vi "FiniteMeasurement.vi"() -> ()   [LabVIEW 2022 SP3]
uses:
  controls/UI References_self.ctl
  <vilib>/Utility/miscctls.llb/LVAnnotationListTypeDef.ctl
  <vilib>/Utility/miscctls.llb/LVCursorListTypeDef.ctl
  controls/Graph Data_self.ctl
  controls/Simulated Signal Type_self.ctl
  controls/HW Configuration_self.ctl
  controls/Analysis Configuration_self.ctl
  controls/New Data Behavior_self.ctl
  controls/User Specified Data_self.ctl
  controls/Data_self.ctl
panel:
  out "状态栏":string
  out "图形":dbl[](graph)
  in  "退出":bool
  in  "导出":bool
  in  "保存":bool
  in  "复制图形":bool
  in  "分析":bool
  in  "清空":bool
  in  "加载":bool
  in  "采集":bool
  in  "设置":bool
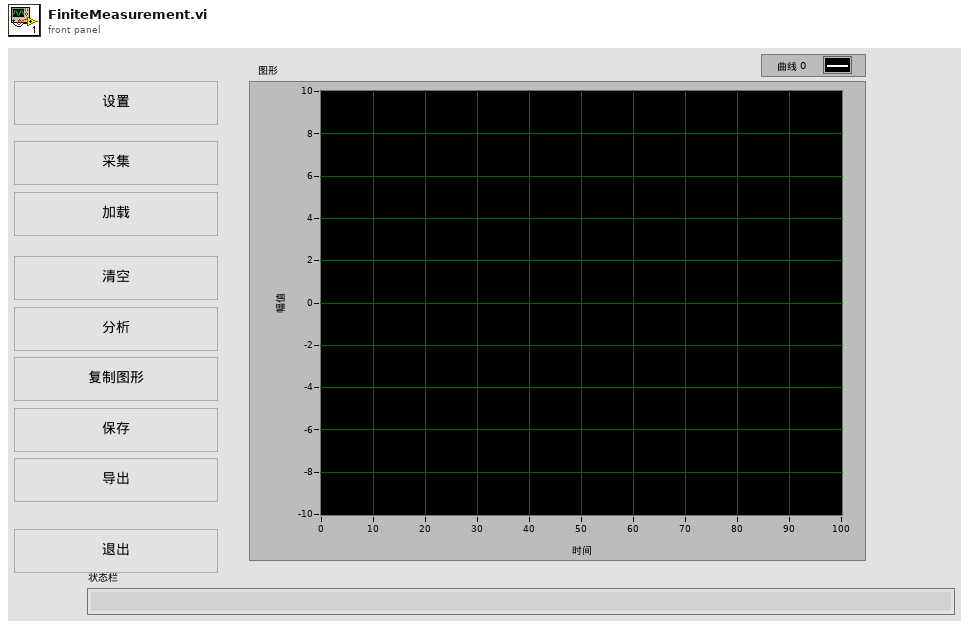
[diagram p1: front panel]
types:
  T1 = typedef "Data_self.ctl" = cluster{"UI引用":T2, "图形数据":T3, "用户定义":T6}
  T2 = typedef "UI References_self.ctl" = cluster{"退出引用":refnum<vi>, "保存引用":refnum<vi>, "打开引用":refnum<vi>, "导出引用":refnum<vi>, "采集引用":refnum<vi>, "配置引用":refnum<vi>, "图形引用":refnum<vi>, "清空引用":refnum<vi>, "分析引用":refnum<vi>, "状态引用":refnum<vi>, "快照引用":refnum<vi>}
  T3 = typedef "Graph Data_self.ctl" = cluster{"数据":waveform(dbl)[], "Annotation List":T4, "Cursor List":T5, "分析数据":waveform(dbl)[]}
  T4 = typedef "LVAnnotationListTypeDef.ctl" = cluster{"Name":string, "Color":u32, "Style":u8, "Point Style":u8, "Name Visible":bool, "Allow Drag":bool, "Annotation Mode":u32, "Plot":i32, "Index":i32, "Position":cluster{"X":dbl, "Y":dbl}, "X Scale":u32, "Y Scale":u32, "Show Arrow":bool, "Lock Name":bool, "Plot Area":i32, "Label Offset":cluster{"X":dbl, "Y":dbl}}[]
  T5 = typedef "LVCursorListTypeDef.ctl" = cluster{"Name":string, "Color":u32, "Style":u8, "Point Style":u8, "Name Visible":bool, "Allow Drag":bool, "Cursor Mode":u32, "Plot":i32, "Index":i32, "Position":cluster{"X":dbl, "Y":dbl}, "X Scale":u32, "Y Scale":u32, "Watch Plots":i32[], "Watch All Plots":bool, "Plot Area":i32, "Label Offset":cluster{"X":dbl, "Y":dbl}}[]
  T6 = typedef "User Specified Data_self.ctl" = cluster{"硬件配置":T7, "分析配置":T9, "新采集到数据时如何操作":T10}
  T7 = typedef "HW Configuration_self.ctl" = cluster{"硬件引用句柄":string, "信号类型":T8}
  T8 = typedef "Simulated Signal Type_self.ctl" = enum16{"Sine Wave", "Square Wave"}
  T9 = typedef "Analysis Configuration_self.ctl" = cluster{"统计":bool}
  T10 = typedef "New Data Behavior_self.ctl" = enum16{"Replace", "Overlay", "Append"}
  T11 = enum16{"Initialize", "Wait for Event", "Update UI", "Configure", "Acquire", "Load Data", "Save Data", "Export Data", "Clear Data", "Analyze", "Copy Graph", "Exit"}
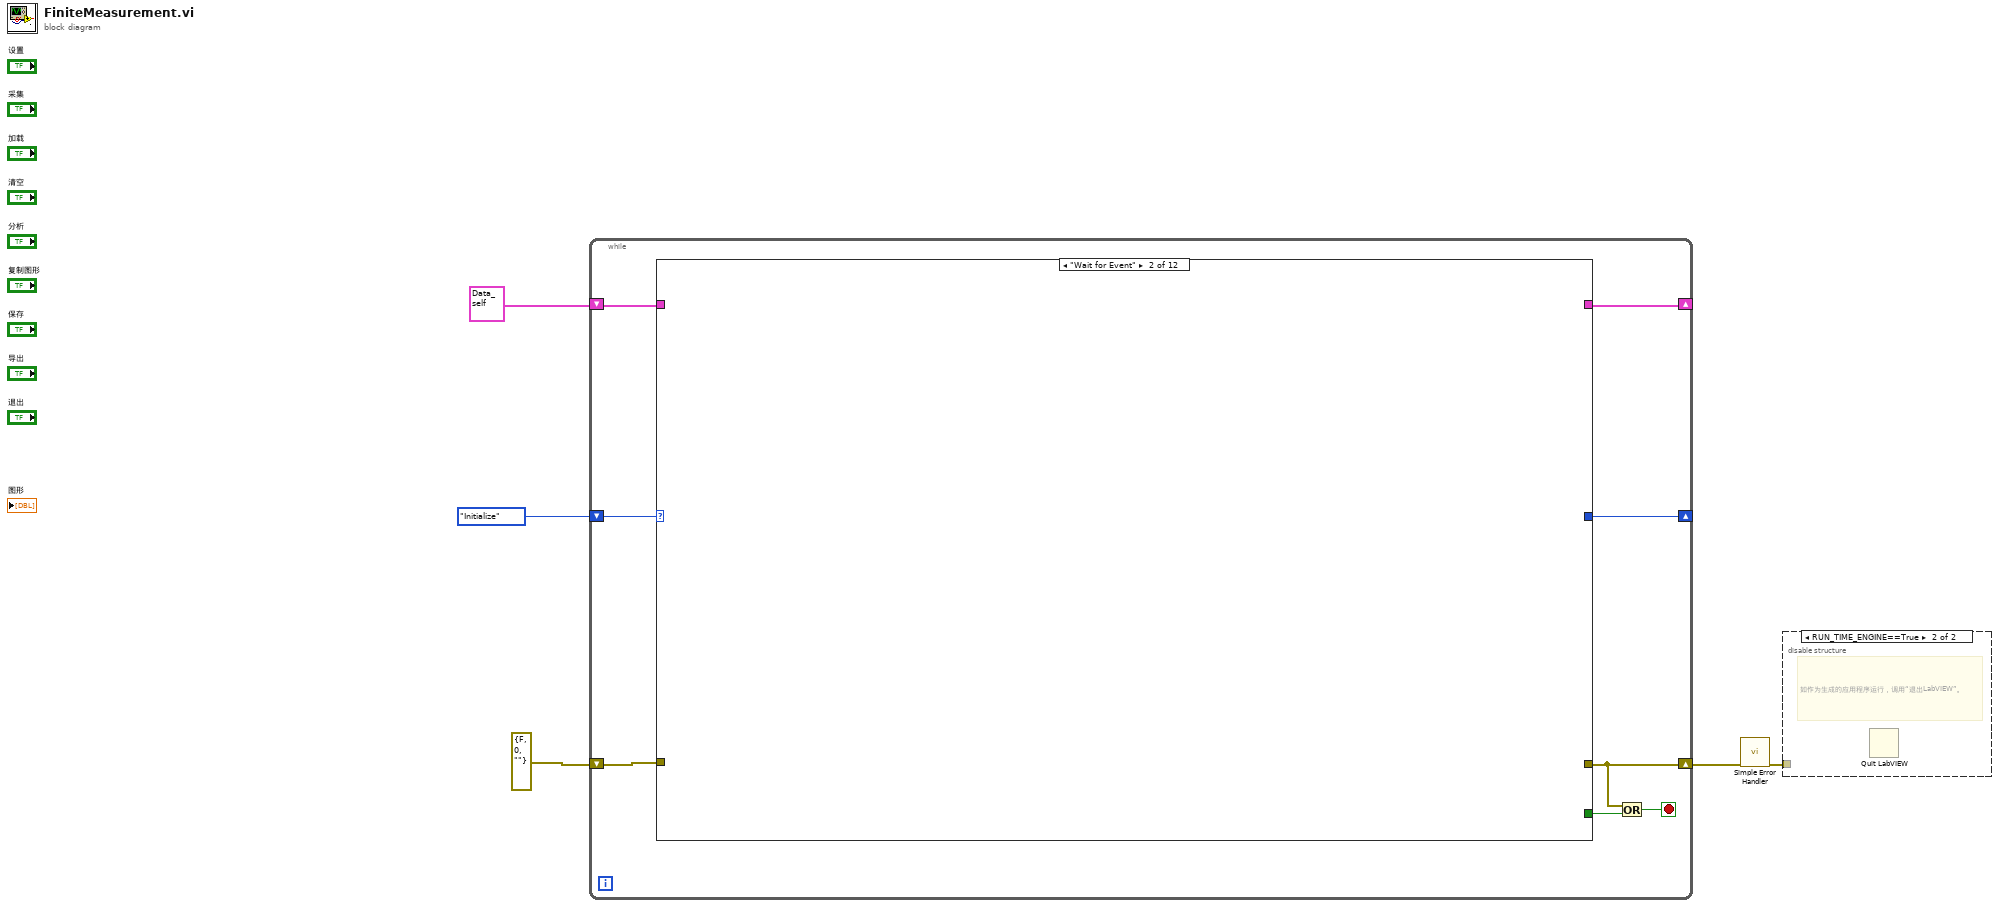
[diagram p0: block diagram]
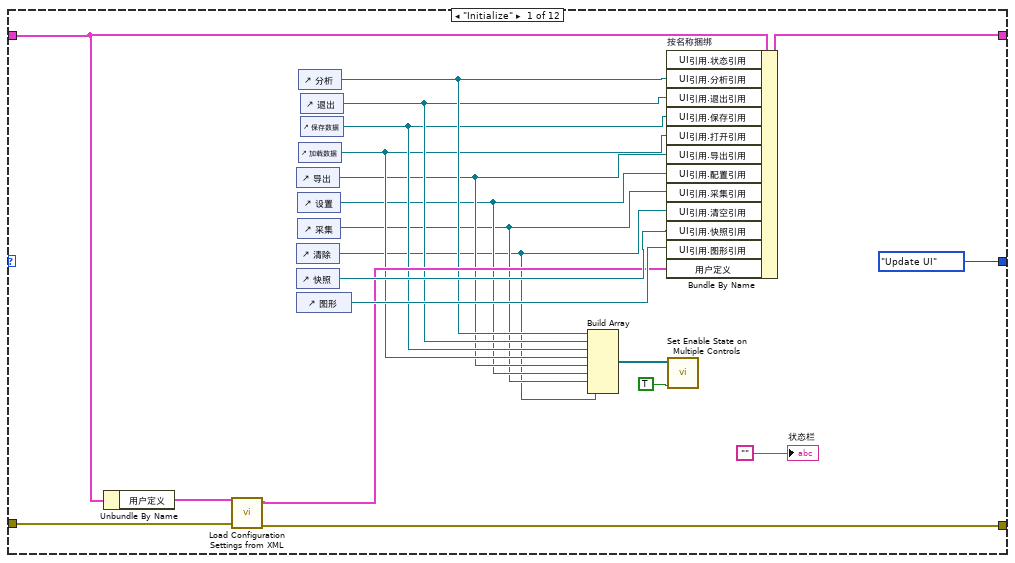
[diagram p3: hidden frame]
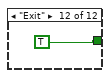
[diagram p13: hidden frame]
diagram:
  n1 = while {
    shift-right: [w10] -> w2
    shift-left: errorcluster {"status"=FALSE, "code"=0, "source"=""} ("错误常量") -> [w12]
    shift-right: [w7] -> _
    shift-left: T1 {"UI引用"={"退出引用"=refnum, "保存引用"=refnum, "打开引用"=refnum, "导出引用"=refnum, "采集引用"=refnum, "配置引用"=refnum, "图形引用"=refnum, "清空引用"=refnum, "分析引用"=refnum, "状态引用"=refnum, "快照引用"=refnum}, "图形数据"={"数据"=[], "Annotation List"=[], "Cursor List"=[], "分析数据"=[]}, "用户定义"={"硬件配置"={"硬件引用句柄"="", "信号类型"=enum."Sine Wave"}, "分析配置"={"统计"=FALSE}, "新采集到数据时如何操作"=enum."Replace"}} ("数据") -> [w8]
    shift-right: [w6] -> _
    shift-left: T11."Initialize" ("枚举") -> [w13]
    stop <- w11 stop-if-true
    n2 = case shown="\"Wait for Event\"" w13 {
      tunnel: w12 -> [w29 _ _ _ w35 _ _ _ _ _ _ _]
      tunnel: [w28 _ _ _ w35 _ _ _ _ _ _ _] -> w10
      tunnel: [_ _ _ _ _ _ _ _ _ _ _ TRUE] -> w9
      tunnel: w8 -> [w34 _ _ _ _ _ _ _ _ _ _ _]
      tunnel: [w33 _ _ _ _ _ _ _ _ _ _ _] -> w7
      tunnel: [T11."Update UI" ("枚举") _ _ _ _ _ _ _ _ _ _ _] -> w6
      frame "Initialize" {
        n3 = Unbundle By Name(w34) -> ("用户定义"=w27:T6)
        n4 = call "Load Configuration Settings from XML.vi"("error in (no error)"=w29, "用户配置输入"=w27) -> ("error out"=w28:errorcluster, "用户配置输出"=w26:T6)  [unwired: 8 in]
        n5 = control-ref of="导出"() -> (w21:refnum<vi>)
        n6 = control-ref of="清除"() -> (w18:refnum<vi>)
        n7 = control-ref of="快照"() -> (w31:refnum<vi>)
        n8 = control-ref of="图形"() -> (w30:refnum<vi>)
        n9 = control-ref of="设置"() -> (w20:refnum<vi>)
        n10 = control-ref of="采集"() -> (w19:refnum<vi>)
        n11 = control-ref of="分析"() -> (w25:refnum<vi>)
        n12 = control-ref of="加载数据"() -> (w22:refnum<vi>)
        n13 = control-ref of="退出"() -> (w24:refnum<vi>)
        n14 = control-ref of="保存数据"() -> (w23:refnum<vi>)
        n15 = Build Array(w25, w24, w23, w22, w21, w20, w19, w18) -> (w17:refnum<vi>[])
        n16 = Bundle By Name "按名称捆绑"(cluster=w34, "UI引用.分析引用"=w25, "UI引用.退出引用"=w24, "UI引用.保存引用"=w23, "UI引用.打开引用"=w22, "UI引用.导出引用"=w21, "UI引用.配置引用"=w20, "UI引用.采集引用"=w19, "UI引用.清空引用"=w18, "UI引用.快照引用"=w31, "UI引用.图形引用"=w30, "用户定义"=w26) -> (w33:T1, "UI引用.状态引用"=w32:refnum<vi>)
        n17 = call "Set Enable State on Multiple Controls.vi"("启用？"=TRUE, "数组"=w17) -> ()  [unwired: 10 in]
        "状态栏" <- ""
      }
      frame "Wait for Event" {
      }
      frame "Update UI" {
      }
      frame "Configure" {
      }
      frame "Acquire" {
      }
      frame "Load Data" {
      }
      frame "Save Data" {
      }
      frame "Export Data" {
      }
      frame "Clear Data" {
      }
      frame "Analyze" {
      }
      frame "Copy Graph" {
      }
      frame "Exit" {
      }
    }
    n18 = Or(x=w10, y=w9) -> (x .or. y?=w11:bool)
  }
  n19 = call <vilib>:"Simple Error Handler.vi"("error in (no error)"=w2) -> ("error out"=w3:errorcluster)  [unwired: 4 in, 4 out]
  n20 = disable-structure "Conditional Disable Structure" shown="RUN_TIME_ENGINE==True" {
    disable-tunnel: w3 -> [_ _]
    frame condition #0 (active) {
    }
    frame condition #1 {
      # "如作为生成的应用程序运行，调用“退出LabVIEW”。"
      n21 = Quit LabVIEW() -> ()  [unwired: 1 in]
    }
  }
